vi "construct.vi"(6 "tablecloth_type":T1 items=["Type 1", "Type 2"], 8 "error in (no error)":errorcluster, 9 "cushion_model":T2 items=["Model 1", "Model 2"], 10 "cost":dbl, 11 "id":u32) -> (0 "error out":errorcluster, 3 "ChairWithTableAttached out":refnum<class "ChairWithTableAttached.lvclass">)   [LabVIEW 2021, in "ChairWithTableAttached.lvclass"]
uses:
  ChairWithTableAttached.lvclass
  IChair/CushionModel.ctl
  ITable/TableclothType.ctl
  ChairWithTableAttached.lvclass/ChairWithTableAttached.ctl
  IChair/IChair.lvclass
  ITable/ITable.lvclass
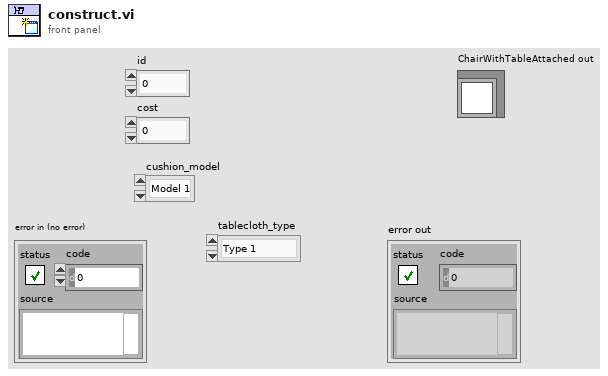
[diagram p1: front panel]
types:
  T1 = typedef "ITable.lvclass/TableclothType.ctl" = u16
  T2 = typedef "IChair.lvclass/CushionModel.ctl" = u16
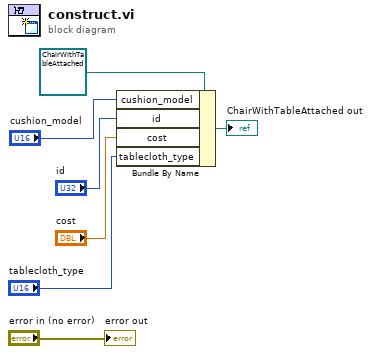
[diagram p0: block diagram]
diagram:
  n1 = Bundle By Name(cluster=refnum<class "ChairWithTableAttached.lvclass"> refnum ("ChairWithTableAttached.lvclass"), "cushion_model"="cushion_model", "id"="id", "cost"="cost", "tablecloth_type"="tablecloth_type") -> (→"ChairWithTableAttached out":refnum<class "ChairWithTableAttached.lvclass">)
  "error out" <- "error in (no error)"
